vi "Calc Time.vi"(8 "error in (no error)":errorcluster, 9 "SP":dbl, 10 "PV":dbl, 11 "ExpFitter in":refnum<class "ExpFitter.lvclass">) -> (0 "error out":errorcluster, 2 "dT":dbl, 3 "ExpFitter out":refnum<class "ExpFitter.lvclass">)   [LabVIEW 2019, in "ExpFitter.lvclass"]
uses:
  ExpFitter.lvclass
  ExpFitter.lvclass/ExpFitter.ctl
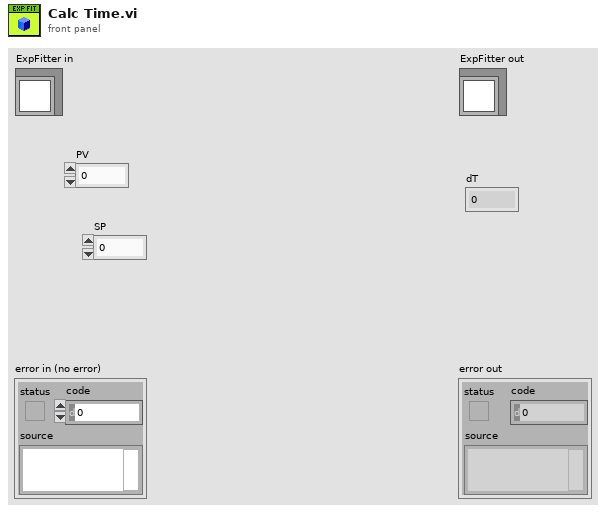
[diagram p1: front panel]
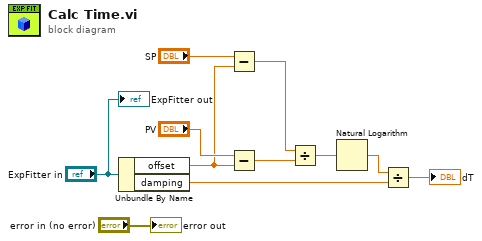
[diagram p0: block diagram]
diagram:
  n1 = Unbundle By Name("ExpFitter in") -> ("offset"=w7:dbl, "damping"=w2:dbl)
  n2 = Subtract(x="SP", y=w7) -> (x-y=w5:dbl)
  n3 = Subtract(x="PV", y=w7) -> (x-y=w6:dbl)
  n4 = Divide(x=w5, y=w6) -> (x/y=w4:dbl)
  n5 = Natural Logarithm(1:w4) -> (0:w3:dbl)
  n6 = Divide(x=w3, y=w2) -> (x/y=→"dT":dbl)
  "error out" <- "error in (no error)"
  "ExpFitter out" <- "ExpFitter in"
